vi "Configure Sequence Repetition Count.vi"(8 "error in (no error)":errorcluster, 9 "Count (1)":i32=1, 10 "Instance (1)":i32=1, 11 "VISA resource name":refnum<visa-resource-name>) -> (0 "error out":errorcluster, 3 "VISA resource name out":refnum<visa-resource-name>)   [LabVIEW 2015, in "Rohde&Schwarz CMXP GPRF.lvlib"]
doc: "Defines how often the sequencer list is processed in SINGle repetition mode.\n\nAttribute(s):\nRSCMXPGPRF_ATTR_SEQUENCE_REPETITION_COUNT\n\nRemote-control command(s):\nSOURce:GPRF:GEN<i>:SEQuencer:NREPetition"
uses:
  <instrlib>/Rohde&Schwarz CMXP GPRF/Rohde&Schwarz CMXP GPRF.lvlib
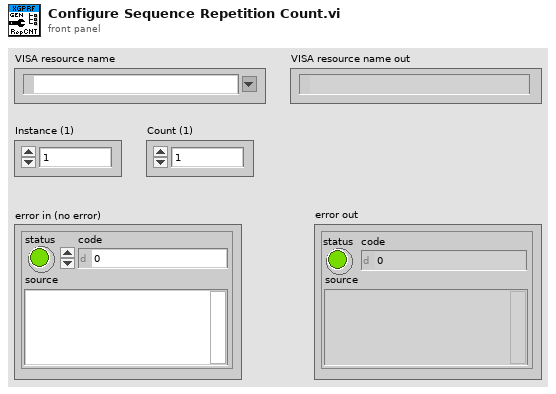
[diagram p1: front panel]
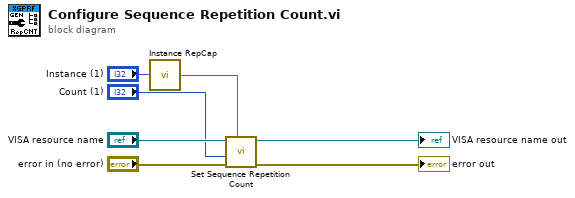
[diagram p0: block diagram]
diagram:
  n1 = call <instrlib>:"Instance RepCap.vi"("instance  in"="Instance (1)") -> ("instance out"=w3:string)
  n2 = call "Set Sequence Repetition Count"("Repeated Capabilities"=w3, "error in (no error)"="error in (no error)", "Sequence Repetition Count (0)"="Count (1)", "instrument handle"="VISA resource name") -> ("error out"=→"error out":errorcluster, "instrument handle out"=→"VISA resource name out":refnum<visa-resource-name>)  [unwired: 6 in]
